vi "TEMOCR-Initialize Data Files.vi"(0 "Expt State":T2, 5 "Params":T3, 7 "State In":T1, 11 "error in (no error)":errorcluster) -> (4 "Run":i32, 8 "State Out":T1, 15 "error out":errorcluster)   [LabVIEW 2015]
uses:
  Typedefs/TEMOCR-Parameters.ctl
  Typedefs/TEMOCR-Probe.ctl
  Typedefs/TEMOCR-Elicitor.ctl
  Human Studies/SFM Frontend/LV Source/Typedefs/HSTS-Transducer.ctl
  Typedefs/TEMOCR-Sequence.ctl
  Typedefs/TEMOCR-Analysis.ctl
  CFTS Main Panel SubVIs/CFTS-Experiment State.ctl
  Typedefs/TEMOCR-Analysis State.ctl
panel:
  in  "TEOAE-MOCR Data File":cluster{"Date":string, "Version":i32}
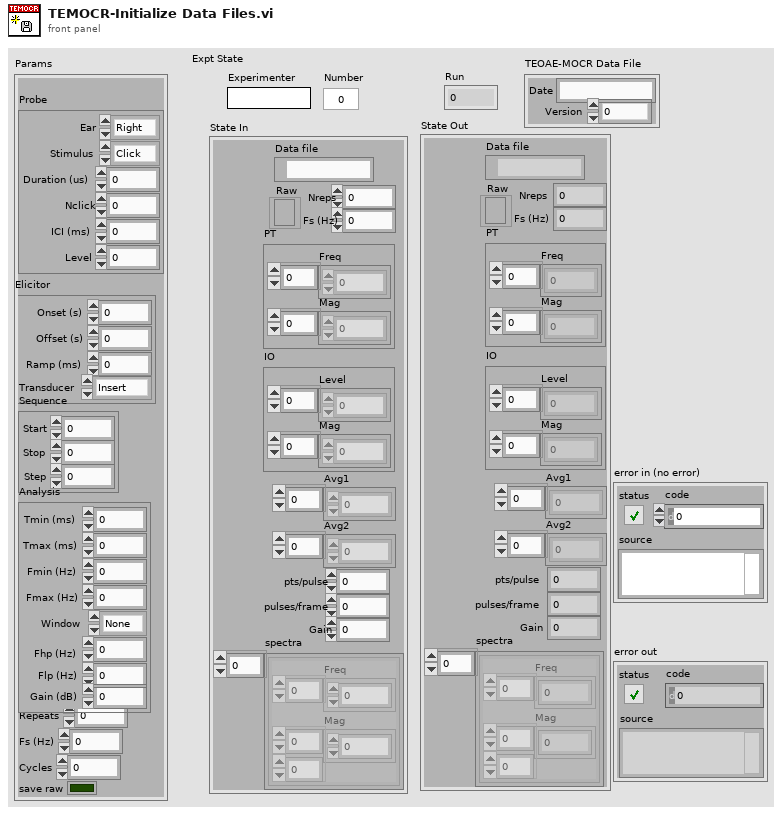
[diagram p1: front panel]
types:
  T1 = typedef "TEMOCR-Analysis State.ctl" = cluster{"Data file":path, "Raw":refnum<file>, "PT":cluster{"Freq":dbl[], "Mag":dbl[]}, "IO":cluster{"Level":dbl[], "Mag":dbl[]}, "Nreps":i32, "Fs (Hz)":dbl, "Avg1":dbl[], "pts/pulse":i32, "pulses/frame":i32, "Avg2":dbl[], "Gain":dbl, "spectra":cluster{"Freq":dbl[], "Mag":dbl[][]}[]}
  T2 = typedef "CFTS-Experiment State.ctl" = cluster{"Experimenter":string, "Number":u32, "Right":string, "Left":string, "Data Folder":path, "State File":path, "Version Info":string, "End Exposure Time":dbl, "Exposure Duration":string, "Run #":cluster{"CAP":i16, "ABR":i16, "DP":i16, "VsEP":i16, "MeasSeq":i16, "SubSeq":i16, "SFOAE":i16}}
  T3 = typedef "TEMOCR-Parameters.ctl" = cluster{"Probe":T4, "Elicitor":T5, "Sequence":T7, "Analysis":T8, "Repeats":i32, "Fs (Hz)":dbl, "Cycles":i32, "save raw":bool}
  T4 = typedef "TEMOCR-Probe.ctl" = cluster{"Ear":enum16{"Right", "Left"}, "Stimulus":enum16{"Click", "Chirp"}, "Duration (us)":dbl, "Nclick":i32, "ICI (ms)":dbl, "Level":dbl}
  T5 = typedef "TEMOCR-Elicitor.ctl" = cluster{"Onset (s)":dbl, "Offset (s)":dbl, "Ramp (ms)":dbl, "Transducer":T6}
  T6 = typedef "HSTS-Transducer.ctl" = enum16{"Insert", "TDH-39", "HD300", "ER-10X"}
  T7 = typedef "TEMOCR-Sequence.ctl" = cluster{"Start":dbl, "Stop":dbl, "Step":dbl}
  T8 = typedef "TEMOCR-Analysis.ctl" = cluster{"Tmin (ms)":dbl, "Tmax (ms)":dbl, "Fmin (Hz)":dbl, "Fmax (Hz)":dbl, "Window":enum16{"None", "Hanning", "Hamming"}, "Fhp (Hz)":dbl, "Flp (Hz)":dbl, "Gain (dB)":dbl}
  T9 = enum16{"open", "replace", "create", "open or create", "replace or create", "replace or create with confirmation"}
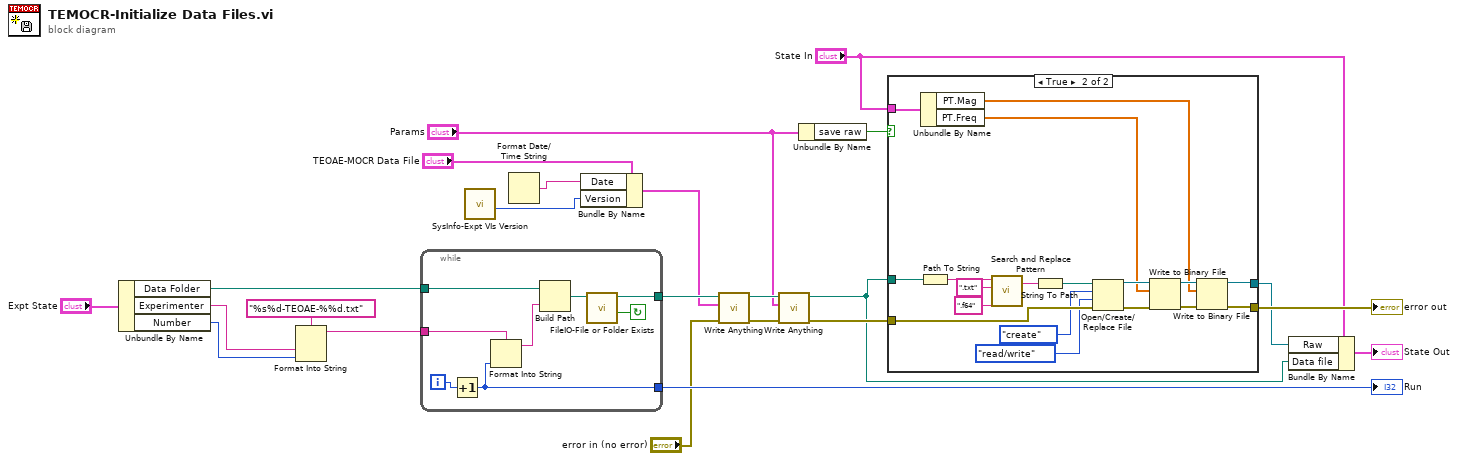
[diagram p0: block diagram]
diagram:
  n1 = Unbundle By Name("Expt State") -> ("Data Folder"=w19:path, "Experimenter"=w21:string, "Number"=w20:u32)
  n2 = Format Into String(format string="%s%d-TEOAE-%%d.txt", w21, w20) -> (resulting string=w18:string)  [unwired: 2 in, 1 out]
  n3 = while {
    tunnel: w19 -> [w29]
    tunnel: w18 -> [w31]
    tunnel: [w25] -> w13
    tunnel: [w24] -> w17
    i -> [w30]
    stop <- w26 continue-if-true
    n4 = Increment(x=w30) -> (x+1=w24:i32)
    n5 = Format Into String(format string=w31, w24) -> (resulting string=w28:string)  [unwired: 2 in, 1 out]
    n6 = Build Path(base path=w29, name or relative path=w28) -> (appended path=w27:path)
    n7 = call "FileIO-File or Folder Exists.vi"("path"=w27) -> ("Exists?"=w26:bool, "dup path"=w25:path)  [unwired: 7 in, 2 out]
  }
  "Run" <- w17
  n8 = call "SysInfo-Expt VIs Version.vi"() -> ("Expt VIs Version out"=w14:i32)  [unwired: 11 in]
  n9 = Format Date/Time String() -> (date/time string=w15:string)  [unwired: 3 in]
  n10 = Bundle By Name(cluster="TEOAE-MOCR Data File", "Date"=w15, "Version"=w14) -> (w12:cluster{"Date":string, "Version":i32})
  n11 = call "Write Anything.vi"("Error In"="error in (no error)", "Anything"=w12, "Path (dialog)"=w13) -> ("Error Out"=w9:errorcluster, "Path out"=w10:path)  [unwired: 7 in]
  n12 = call "Write Anything.vi"("Error In"=w9, "Anything"="Params", "Path (dialog)"=w10) -> ("Error Out"=w6:errorcluster, "Path out"=w2:path)  [unwired: 7 in]
  n13 = Unbundle By Name("Params") -> ("save raw"=w7:bool)
  n14 = case shown="True" w7 {
    tunnel: w2 -> [_ w50]
    tunnel: w6 -> [w32 w44]
    tunnel: [_ w34] -> w3
    tunnel: [w32 w33] -> w5
    tunnel: "State In" -> [_ w41]
    frame False {
    }
    frame True {
      n15 = Path To String(path=w50) -> (string=w49:string)
      n16 = Unbundle By Name(w41) -> ("PT.Mag"=w35:dbl[], "PT.Freq"=w38:dbl[])
      n17 = call <vilib>:"Search and Replace Pattern.vi"("string"=w49, "regular expression (\"\")"=".txt" ("regular expression (\"\")"), "replace string (\"\")"=".f64" ("replace string (\"\")")) -> ("result string"=w46:string)  [unwired: 2 in, 1 out]
      n18 = String To Path(string=w46) -> (path=w45:path)
      n19 = Open/Create/Replace File(file path (use dialog)=w45, error in=w44, operation (0:open)=T9."create", access (0:read/write)=enum16{"read/write", "read-only", "write-only"}."read/write") -> (refnum out=w39:refnum<file>, error out=w40:errorcluster)  [unwired: 2 in, 1 out]
      n20 = Write to Binary File(file (use dialog)=w39, data=w38, error in=w40) -> (refnum out=w36:refnum<file>, error out=w37:errorcluster)  [unwired: 3 in, 1 out]
      n21 = Write to Binary File(file (use dialog)=w36, data=w35, error in=w37) -> (refnum out=w34:refnum<file>, error out=w33:errorcluster)  [unwired: 3 in, 1 out]
    }
  }
  "error out" <- w5
  n22 = Bundle By Name(cluster="State In", "Raw"=w3, "Data file"=w2) -> (→"State Out":T1)
